vi "George.vi"() -> ()   [LabVIEW 2014]
uses:
  <userlib>/CurtinCode/DataControl.ctl
  <userlib>/CurtinCode/SettingsControl.ctl
  <userlib>/CurtinCode/FilterCtrl.ctl
  <vilib>/sound2/lvsound2.llb/Sound File Info (path).vi
panel:
  out "Average FRF":cluster{dbl, "df":dbl, dbl[]}
  in  "Filter":T1 items=["None", "1 Octave", "1/3 Octave", "1/12 Octave", "Custom"]
  in  "Delete last Run":bool
  out "Average":string
  out "Pts in Ave":u8
  out "selected paths":path[](array[path])
  in  "Open File":bool
  out "Mic Spectrum":cluster{dbl, "df":dbl, dbl[]}(graph)
  out "Alarm":string
  out "Raw Data":T2={"Settings"={"Data Path"=path "", "Time"=timestamp(0 s since 1904-01-01), "Sampling Rate (Hz)"=44800, "Device"=0, "pre-trigger (sec)"=100.0, "length of sample (sec)"=1000.0, "trigger value (V)"=100.0, "Labels"=[], "Cutoffs (sec)"=[], "Freq Bands"=[]}, "Data"=[], "Plot type"=enum."Linear"} {"Settings"."Time" format="%<%H:%M\n%d/%m/%y>T"}
  in  "Tab Control":enum32{"Page 1", "Page 2"}(tab)
  in  "Close Help":bool
  out "Help Text":bool
  in  "Help":bool
  out "version":string="0.1"
  in  "Test":bool
  out "Point":u8(slide) scale=0.0..12.0
  out "Hit":u8(slide) scale=0.0..5.0
  out "current run":string
  in  "Run Conditions":T4={"hits per point"=5, "points per run"=12, "Project Path"=path ""} {"hits per point" items=["1 hit/pt"=1, "5 hits/pt"=5, "10 hits/pt"=10]; "points per run" items=["1 pt/run"=1, "6 pts/run"=6, "12 pts/run"=12]}
  in  "Record":bool
  in  "microphone settings":T5={"resolution"=24, "Sampling rate"=44100, "Sample time"=1.0, "device"=0} {"device" items=["Microphone (High Definition Audio Device)"=0, "DAQmx"=1000]; "resolution" items=["16 bit"=16, "24 bit"=24, "32 bit"=32]; "Sample time" items=["0.5 s"=0.5, "1 s"=1.0]; "Sampling rate" items=["22050 samp/s"=22050, "44100 samp/s"=44100, "48000 samp/s"=48000]}
  out "Filtered FRF":cluster{"Fctr":ext[], "magnitude":dbl[]}[](graph)
  out "Hammer":cluster{i32, dbl, "Data set":dbl[]}(graph)
  out "Microphone":cluster{i32, dbl, "Data set":dbl[]}(graph)
  out "Hammer spectrum":cluster{dbl, "df":dbl, dbl[]}(graph)
  out "Current FRF":cluster{dbl, "df":dbl, dbl[]}(graph)
  out "Live Mic":cluster{i32, dbl, "Data set":dbl[]}(graph)
  # "The Violin Analyzer - version"
  # "Run a test or record an entire run"
  # "See Progess through run"
  # "Set cutoff with green cursors"
  # "Set threshold with purple cursor"
  # "Select Input Device and Settings"
  # "Name Run and Set Run Parameters"
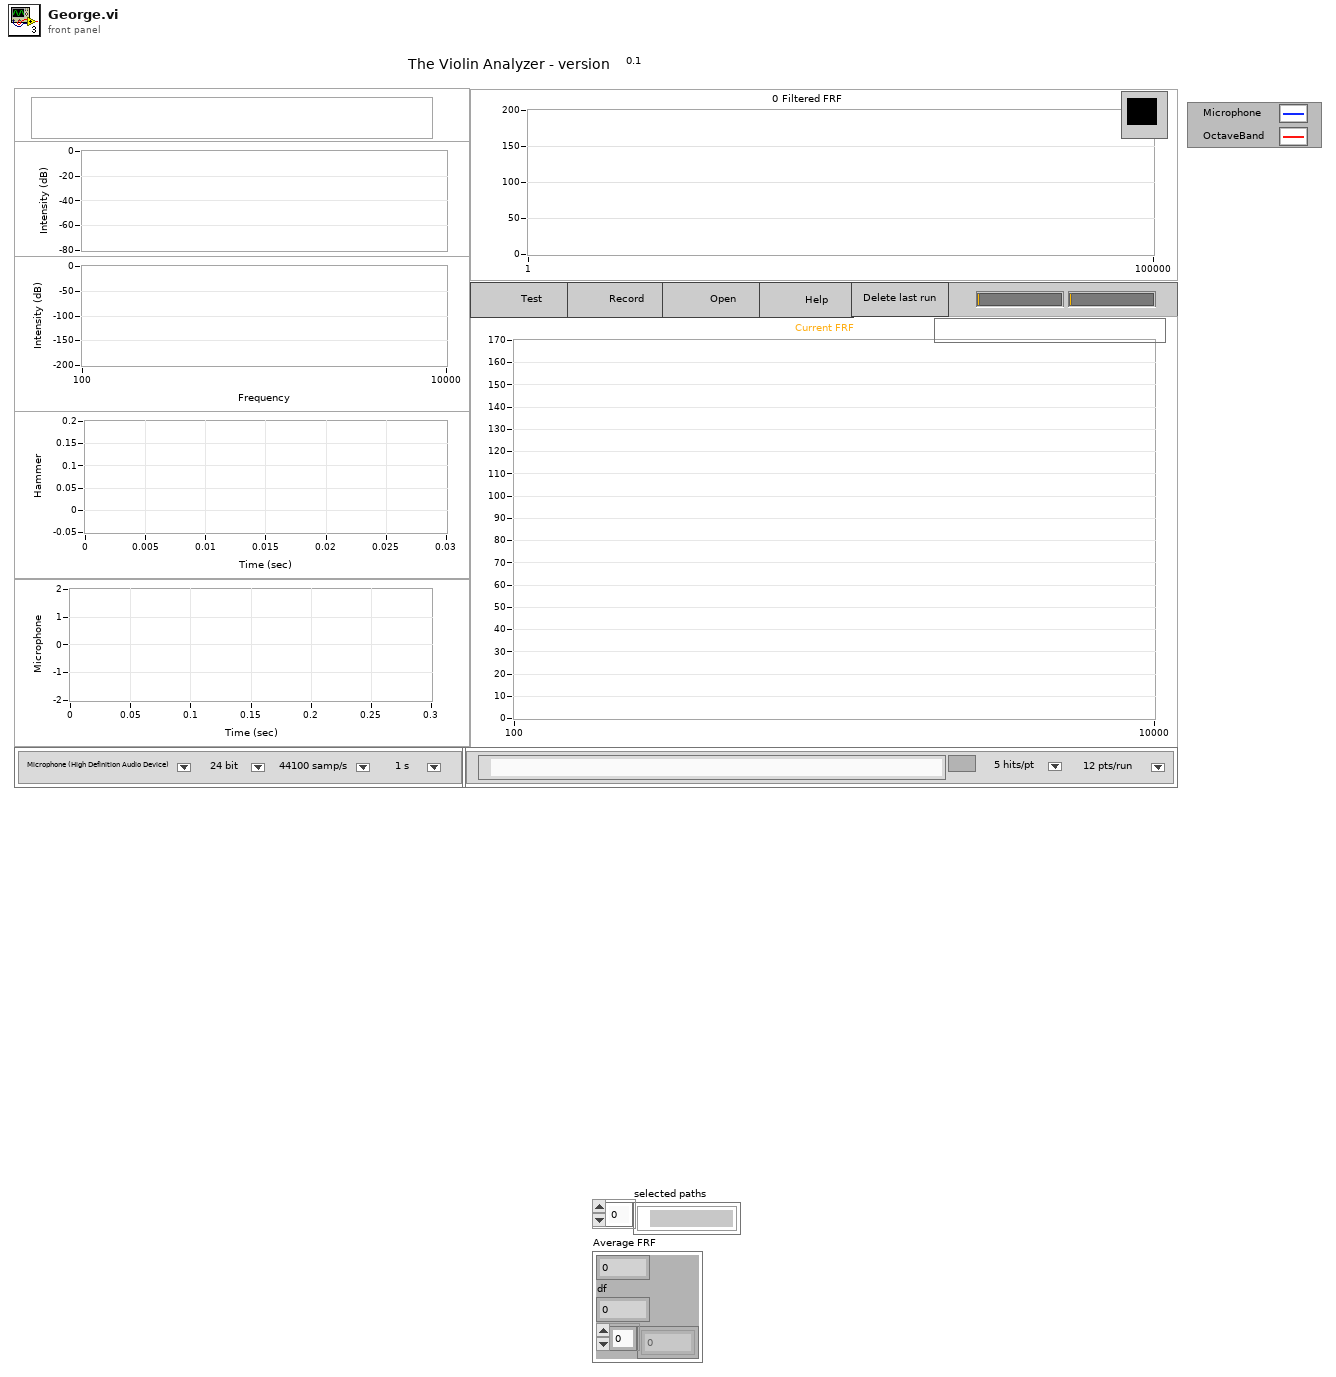
[diagram p1: front panel]
types:
  T1 = typedef "FilterCtrl.ctl" = i8
  T2 = typedef "DataControl.ctl" = cluster{"Settings":T3, "Data":cluster{i32, dbl, "data":dbl[]}[], "Plot type":enum16{"Linear", "log"}}
  T3 = typedef "SettingsControl.ctl" = cluster{"Data Path":path, "Time":timestamp, "Sampling Rate (Hz)":u16, "Device":u16, "pre-trigger (sec)":dbl, "length of sample (sec)":dbl, "trigger value (V)":dbl, "Labels":string[], "Cutoffs (sec)":dbl[], "Freq Bands":dbl[]}
  T4 = cluster{"hits per point":u16, "points per run":u16, "Project Path":path}
  T5 = cluster{"resolution":u16, "Sampling rate":u16, "Sample time":dbl, "device":u16}
  T6 = typedef "AllDataCtrl.ctl" = cluster{"Data Set":T2, "number of samples/ch":i32, "task ID":T7, "error out":errorcluster, "DAQmx task":refnum<k21>}
  T7 = typedef "Sound Input Task ID.ctl" = u32
  T8 = typedef "Sound Data Format.ctl" = cluster{"sample rate (S/s)":dbl, "number of channels":i32, "bits per sample":i32}
  T9 = typedef "LVRangeTypeDef.ctl" = cluster{"Minimum":dbl, "Maximum":dbl, "Increment":dbl, "Minor Increment":dbl, "Start":dbl}
  T10 = typedef "LVStringsAndValuesArrayTypeDef.ctl" = cluster{"String":string, "Value":ext}[]
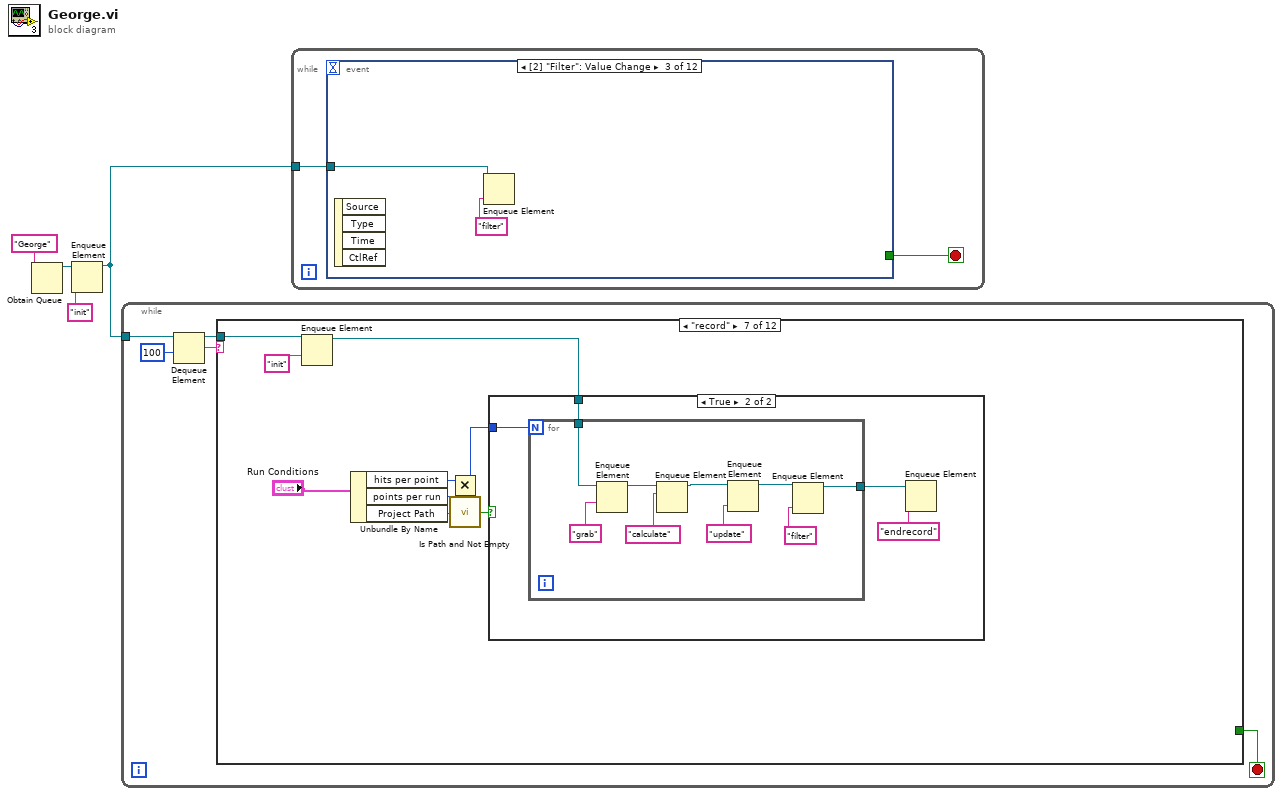
[diagram p0: block diagram]
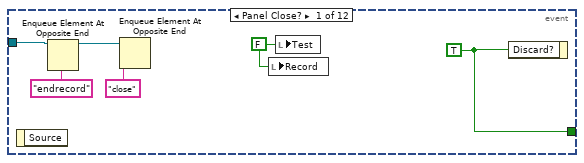
[diagram p2: hidden frame]
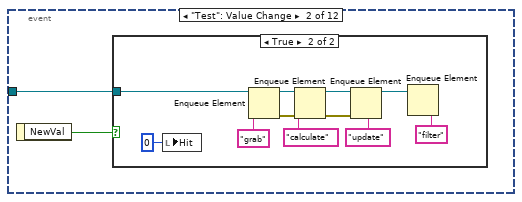
[diagram p3: hidden frame]
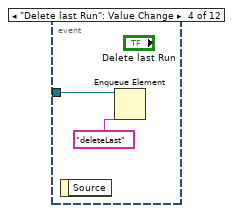
[diagram p5: hidden frame]
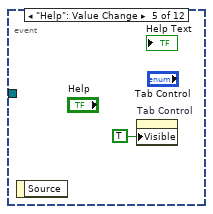
[diagram p6: hidden frame]
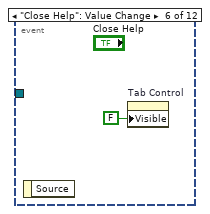
[diagram p7: hidden frame]
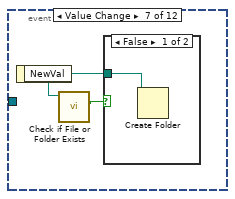
[diagram p8: hidden frame]
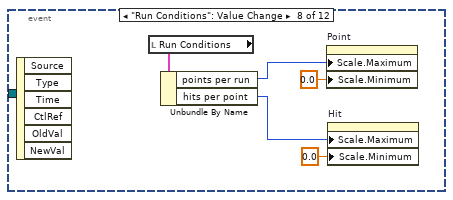
[diagram p10: hidden frame]
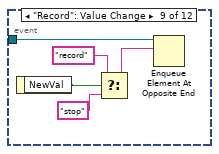
[diagram p11: hidden frame]
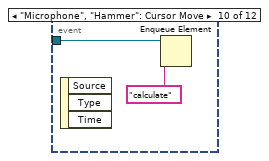
[diagram p12: hidden frame]
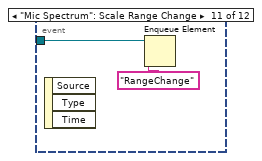
[diagram p13: hidden frame]
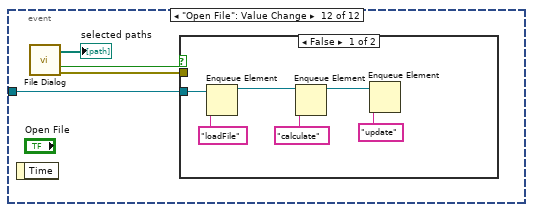
[diagram p14: hidden frame]
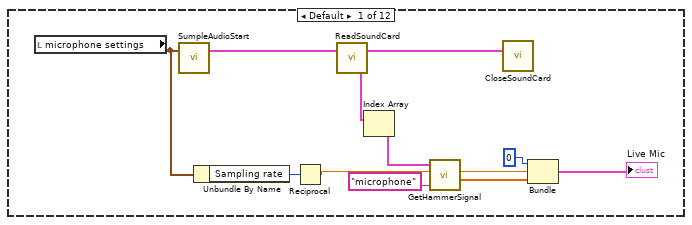
[diagram p16: hidden frame]
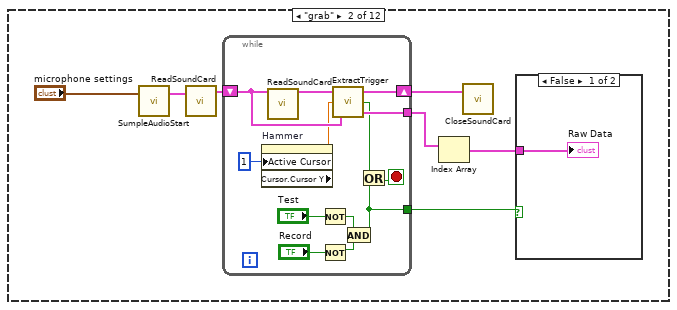
[diagram p17: hidden frame]
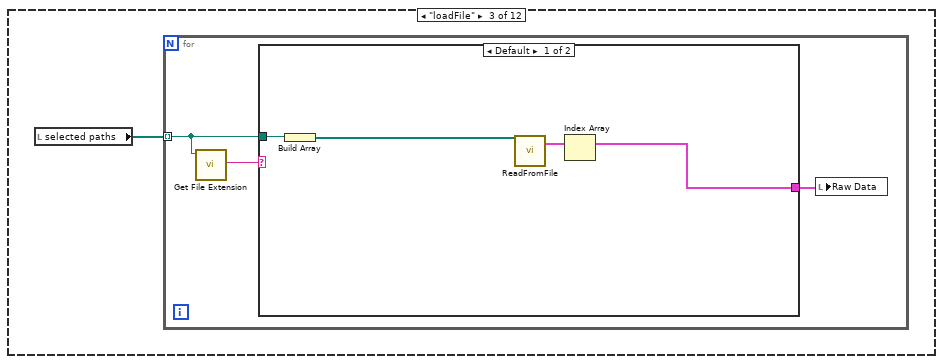
[diagram p19: hidden frame]
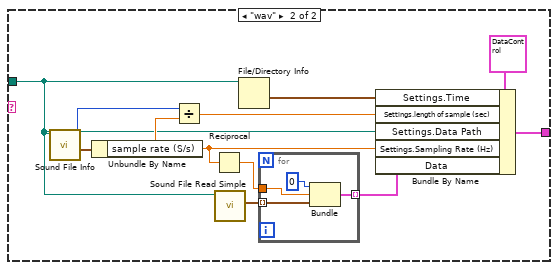
[diagram p20: hidden frame]
diagram:
  w4 = "George" ("name (unnamed)")
  n1 = Obtain Queue(name (unnamed)=w4, element data type=w4) -> (queue out=w3:refnum<queue>)  [unwired: 3 in, 2 out]
  n2 = Enqueue Element(queue=w3, element="init") -> (queue out=w1:refnum<queue>)  [unwired: 2 in, 2 out]
  n3 = while {
    tunnel: w1 -> [w9]
    stop <- w7 stop-if-true
    n4 = Dequeue Element(queue=w9, timeout in ms (-1)=100) -> (queue out=w6:refnum<queue>, element=w8:string)  [unwired: 1 in, 2 out]
    n5 = case shown="\"record\"" w8 {
      tunnel: [_ _ _ _ _ _ _ _ _ _ _ TRUE ("Discard?")] -> w7
      tunnel: w6 -> [_ _ _ _ _ _ w156 _ w178 _ w225 _]
      frame Default {
        n6 = local read "microphone settings"() -> (w12:T5)
        n7 = call <userlib>:"SumpleAudioStart.vi"("microphone settings"=w12) -> ("All Info"=w20:T6)  [unwired: 2 in]
        n8 = Unbundle By Name(w12) -> ("Sampling rate"=w13:u16)
        n9 = Reciprocal(x=w13) -> (1/x=w11:dbl)
        n10 = call <userlib>:"ReadSoundCard.vi"("All Info"=w20) -> ("Data Set"=w18:T2[], "All Info"=w19:T6)  [unwired: 1 in]
        n11 = Index Array(array=w18) -> (element=w17:T2)  [unwired: 1 in]
        n12 = call <userlib>:"GetHammerSignal.vi"("column"="microphone", "Data Set"=w17) -> ("Data set"=w14:dbl[])  [unwired: 1 in, 2 out]
        n13 = call <userlib>:"CloseSoundCard.vi"("All Info"=w19) -> ()  [unwired: 3 in]
        n14 = Bundle(0, w11, "Data set"=w14) -> (→"Live Mic":cluster{i32, dbl, "Data set":dbl[]})  [unwired: 1 in]
      }
      frame "grab" {
        n15 = call <userlib>:"SumpleAudioStart.vi"("microphone settings"="microphone settings") -> ("All Info"=w26:T6)  [unwired: 2 in]
        n16 = call <userlib>:"ReadSoundCard.vi"("All Info"=w26) -> ("All Info"=w25:T6)  [unwired: 1 in, 1 out]
        n17 = while {
          shift-right: [w41] -> w27
          shift-left: w25 -> [w39]
          tunnel: [w38] -> w23
          tunnel: [w29] -> w21
          stop <- w33 stop-if-true
          n18 = property on="Hammer" class="WFGraph (strict)"("Active Cursor"=u32 1) -> ("Cursor.Cursor Y"=w36:dbl)  [unwired: 2 in, 2 out]
          n19 = call <userlib>:"ReadSoundCard.vi"("All Info"=w39) -> ("All Info"=w40:T6)  [unwired: 1 in, 1 out]
          n20 = Not(x="Test") -> (.not. x?=w30:bool)
          n21 = Not(x="Record") -> (.not. x?=w31:bool)
          n22 = call <userlib>:"ExtractTrigger.vi"(3:"All Info"=w39, "Trigger"=w36, 5:"All Info"=w40) -> ("Data Set"=w38:T2[], "Trigger?"=w35:bool, "All Info"=w41:T6)
          n23 = And(x=w30, y=w31) -> (x .and. y?=w29:bool)
          n24 = Or(x=w35, y=w29) -> (x .or. y?=w33:bool)
        }
        n25 = Index Array(array=w23) -> (element=w22:T2)  [unwired: 1 in]
        n26 = call <userlib>:"CloseSoundCard.vi"("All Info"=w27) -> ()  [unwired: 3 in]
        n27 = case shown="False" w21 {
          tunnel: w22 -> [w28 _]
          frame False {
            "Raw Data" <- w28
          }
          frame True {
          }
        }
      }
      frame "loadFile" {
        n28 = local read "selected paths"() -> (w42:path[])
        n29 = for {
          tunnel: w42 -> [w44] mode=indexing
          n30 = call <vilib>:"Get File Extension.vi"("file"=w44) -> ("lowercase file extension"=w43:string)  [unwired: 7 in, 3 out]
          n31 = case shown="Default" w43 {
            tunnel: [w46 w52] -> w45
            tunnel: w44 -> [w49 w50]
            frame Default {
              n32 = Build Array(w49) -> (w48:path[])
              n33 = call <userlib>:"ReadFromFile.vi"("File paths"=w48) -> ("Data Sets"=w47:T2[])  [unwired: 1 in, 1 out]
              n34 = Index Array(array=w47) -> (element=w46:T2)  [unwired: 1 in]
            }
            frame "wav" {
              n35 = call-poly <vilib>:"Sound File Info.vi"("path"=w50) -> ("sound format"=w59:T8, "total number of samples/ch"=w55:u32)  [unwired: 7 in, 2 out]
              n36 = Unbundle By Name(w59) -> ("sample rate (S/s)"=w56:dbl)
              n37 = Divide(x=w55, y=w56) -> (x/y=w54:dbl)
              n38 = Reciprocal(x=w56) -> (1/x=w60:dbl)
              n39 = call <vilib>:"Sound File Read Simple.vi"("path"=w50) -> ("data"=w57:waveform(dbl)[])  [unwired: 7 in, 3 out]
              n40 = File/Directory Info(path=w50) -> (last mod=w53:timestamp)  [unwired: 1 in, 6 out]
              n41 = for {
                tunnel: w60 -> [w63]
                tunnel: [w62] -> w58 mode=indexing
                tunnel: w57 -> [w61] mode=indexing
                n42 = Bundle(0, w63, "data"=w61) -> (w62:cluster{i32, dbl, "data":waveform(dbl)})  [unwired: 1 in]
              }
              n43 = Bundle By Name(cluster=T2 {"Settings"={"Data Path"=path "", "Time"=timestamp(0 s since 1904-01-01), "Sampling Rate (Hz)"=44800, "Device"=0, "pre-trigger (sec)"=100.0, "length of sample (sec)"=1000.0, "trigger value (V)"=100.0, "Labels"=[], "Cutoffs (sec)"=[], "Freq Bands"=[]}, "Data"=[], "Plot type"=enum."Linear"} ("Data Set"), "Settings.Time"=w53, "Settings.length of sample (sec)"=w54, "Settings.Data Path"=w50, "Settings.Sampling Rate (Hz)"=w56, "Data"=w58) -> (w52:T2)
            }
          }
          n44 = local write "Raw Data"(w45) -> ()
        }
      }
      frame "calculate" {
        n45 = property on="Hammer" class="WFGraph (strict)"("Active Cursor"=u32 0) -> ("Cursor.Cursor X"=w69:dbl)  [unwired: 2 in, 2 out]
        n46 = property on="Microphone" class="WFGraph (strict)"("Active Cursor"=u32 0) -> ("Cursor.Cursor X"=w70:dbl)  [unwired: 2 in, 2 out]
        n47 = Build Array(w70, w69) -> (w71:dbl[])
        n48 = local read "Raw Data"() -> (w92:T2)
        n49 = Bundle By Name(cluster=w92, "Settings.Cutoffs (sec)"=w71) -> (w68:T2)
        n50 = local read "microphone settings"() -> (w91:T5)
        n51 = Unbundle By Name(w91) -> ("Sampling rate"=w90:u16)
        n52 = local write "Raw Data"(w68) -> ()
        n53 = Reciprocal(x=w90) -> (1/x=w88:dbl)
        n54 = call <userlib>:"GetHammerSignal.vi"("column"="hammer", "Data Set"=w68) -> ("Cutoff"=w94:dbl, "Data set"=w86:dbl[], "time between samples"=w93:dbl)  [unwired: 1 in]
        n55 = call <userlib>:"GetHammerSignal.vi"("column"="microphone", "Data Set"=w68) -> ("Cutoff"=w96:dbl, "Data set"=w81:dbl[], "time between samples"=w97:dbl)  [unwired: 1 in]
        n56 = Bundle(0, w88, "Data set"=w86) -> (→"Hammer":cluster{i32, dbl, "Data set":dbl[]})  [unwired: 1 in]
        n57 = call <userlib>:"FourierTransform.vi"("Cutoff (s)"=w94, "Time Data"=w86, "time per sample"=w93) -> ("Spectrum"=→"Hammer spectrum":cluster{dbl, "df":dbl, dbl[]}, "FFT"=w67:cluster{dbl, "df":dbl, "FFT {X}":cdb[]})
        n58 = Bundle(0, w88, "Data set"=w81) -> (→"Microphone":cluster{i32, dbl, "Data set":dbl[]})  [unwired: 1 in]
        n59 = call <userlib>:"FourierTransform.vi"("Cutoff (s)"=w96, "Time Data"=w81, "time per sample"=w97) -> ("Spectrum"=→"Mic Spectrum":cluster{dbl, "df":dbl, dbl[]}, "FFT"=w66:cluster{dbl, "df":dbl, "FFT {X}":cdb[]})
        n60 = Greater?(x=w81, y=0.99) -> (0:w83:bool[])
        n61 = Greater?(x=w86, y=0.99) -> (0:w84:bool[])
        n62 = call <userlib>:"FindFRF.vi"("Microphone FFT"=w66, "Hammer FFT"=w67) -> ("Current FRF"=→"Current FRF":cluster{dbl, "df":dbl, dbl[]})  [unwired: 1 out]
        n63 = Or Array Elements(Boolean array=w83) -> (logical OR=w80:bool)
        n64 = Or Array Elements(Boolean array=w84) -> (logical OR=w77:bool)
        n65 = Select(t="Microphone Signal Clipped", s=w80, f="") -> (s? t:f=w76:string)
        n66 = Select(t="Hammer Signal Clipped", s=w77, f=w76) -> (s? t:f=w74:string)
        n67 = local write "Alarm"(w74) -> ()
      }
      frame "RangeChange" {
        n68 = property on="Mic Spectrum" class="WFGraph (strict)"() -> (error out=w104:errorcluster, "XScale.Range"=w103:T9)  [unwired: 2 in, 1 out]
        n69 = property on="Hammer spectrum" class="WFGraph (strict)"(error in=w104, "XScale.Range"=w103) -> ()  [unwired: 1 in, 2 out]
      }
      frame "init" {
        w105 = FALSE ("Test")
        w130 = u8 0 ("% done for run")
        w111 = "" ("current run")
        n70 = local read "Run Conditions"() -> (w107:T4)
        n71 = Unbundle By Name(w107) -> ("points per run"=w109:u16, "hits per point"=w106:u16)
        n72 = flat-sequence {
          tunnel: [w131] -> _
          frame #0 {
            n73 = control-ref of="device"() -> (w138:refnum<vi>)
            n74 = call <vilib>:"InitializeInputDeviceRing.vi"("Device Refnum"=w138) -> ("error out"=w137:errorcluster)  [unwired: 1 in, 13 out]
            n75 = property class="Ring (strict)"(reference=w138, error in=w137) -> (reference out=w133:refnum<vi>, error out=w132:errorcluster, "Strings And Values []"=w136:T10)
            n76 = Build Array (concatenate)(w136, cluster{"String":string, "Value":i32} {"String"="DAQmx", "Value"=1000}) -> (w134:T10)
            n77 = property class="Ring (strict)"(reference=w133, error in=w132, "Strings And Values []"=w134) -> (error out=w131:errorcluster)  [unwired: 1 out]
          }
        }
        n78 = property on="Point" class="Slide (strict)"("Scale.Maximum"=w109, "Scale.Minimum"=0.0 ("Scale.Range:Minimum")) -> ()  [unwired: 2 in, 2 out]
        n79 = property on="Hit" class="Slide (strict)"("Scale.Maximum"=w106, "Scale.Minimum"=0.0 ("Scale.Range:Minimum")) -> ()  [unwired: 2 in, 2 out]
        n80 = property on="Tab Control" class="TabCtl (strict)"("Visible"=FALSE) -> ()  [unwired: 2 in, 2 out]
        n81 = local write "Record"(w105) -> ()
        n82 = local write "current run"(w111) -> ()
        n83 = local write "Test"(w105) -> ()
        n84 = local write "Average"(w111) -> ()
        n85 = property on="Hammer" class="WFGraph (strict)"("Active Cursor"=u32 1) -> ("Cursor.Cursor Y"=w114:dbl, "YScale.Maximum"=w112:dbl)  [unwired: 2 in, 2 out]
        n86 = property on="Hammer" class="WFGraph (strict)"("Active Cursor"=u32 0) -> ("Cursor.Cursor X"=w115:dbl, "XScale.Maximum"=w113:dbl)  [unwired: 2 in, 2 out]
        n87 = property on="Microphone" class="WFGraph (strict)"("Active Cursor"=u32 0) -> ("Cursor.Cursor X"=w127:dbl, "XScale.Maximum"=w126:dbl)  [unwired: 2 in, 2 out]
        n88 = In Range and Coerce(upper limit=0.0, x=w114, lower limit=w112) -> (In Range?=w117:bool)  [unwired: 1 out]
        n89 = In Range and Coerce(upper limit=0.0, x=w115, lower limit=w113) -> (In Range?=w118:bool)  [unwired: 1 out]
        n90 = In Range and Coerce(upper limit=0.0, x=w127, lower limit=w126) -> (In Range?=w124:bool)  [unwired: 1 out]
        n91 = And(x=w118, y=w117) -> (x .and. y?=w116:bool)
        n92 = case shown="False" w124 {
          frame False {
            n93 = property on="Microphone" class="WFGraph (strict)"("Active Cursor"=u32 0, "Cursor.Cursor X"=0.2 ("Cursor.Cursor Position:Cursor X")) -> ()  [unwired: 2 in, 2 out]
          }
          frame True {
          }
        }
        n94 = case shown="False" w116 {
          tunnel: w113 -> [w144 _]
          tunnel: w112 -> [w140 _]
          frame False {
            n95 = Divide(x=w144, y=2.0 ("upper limit")) -> (x/y=w142:dbl)
            n96 = Divide(x=w140, y=2.0 ("upper limit")) -> (x/y=w139:dbl)
            n97 = property on="Hammer" class="WFGraph (strict)"("Active Cursor"=u32 0, "Cursor.Cursor X"=w142, "Active Cursor"=u32 1, "Cursor.Cursor Y"=w139) -> ()  [unwired: 2 in, 2 out]
          }
          frame True {
          }
        }
        "Point" <- w130
        "Hit" <- w130
        "version" <- "0.1" ("version")
        "Alarm" <- w111
      }
      frame "record" {
        n98 = Enqueue Element(queue=w156, element="init") -> (queue out=w150:refnum<queue>)  [unwired: 2 in, 2 out]
        n99 = Unbundle By Name("Run Conditions") -> ("hits per point"=w153:u16, "points per run"=w152:u16, "Project Path"=w155:path)
        n100 = Multiply(x=w153, y=w152) -> (x*y=w151:u16)
        n101 = call <vilib>:"Is Path and Not Empty.vi"("path"=w155) -> ("Is Path and Not Empty?"=w154:bool)  [unwired: 4 in]
        n102 = case shown="True" w154 {
          tunnel: w151 -> [_ w163]
          tunnel: w150 -> [_ w162]
          frame False {
            n103 = One Button Dialog(message="Please choose a folder for data") -> ()  [unwired: 1 in, 1 out]
            n104 = local write "Record"(FALSE ("Record")) -> ()
          }
          frame True {
            n105 = for {
              N: w163 -> [_]
              tunnel: w162 -> [w171]
              tunnel: [w164] -> w161
              n106 = Enqueue Element(queue=w171, element="grab") -> (queue out=w169:refnum<queue>)  [unwired: 2 in, 2 out]
              n107 = Enqueue Element(queue=w169, element="calculate") -> (queue out=w168:refnum<queue>)  [unwired: 2 in, 2 out]
              n108 = Enqueue Element(queue=w168, element="update") -> (queue out=w165:refnum<queue>)  [unwired: 2 in, 2 out]
              n109 = Enqueue Element(queue=w165, element="filter") -> (queue out=w164:refnum<queue>)  [unwired: 2 in, 2 out]
            }
            n110 = Enqueue Element(queue=w161, element="endrecord") -> ()  [unwired: 2 in, 3 out]
          }
        }
      }
      frame "endrecord" {
        w173 = "" ("Alarm")
        n111 = local write "Test"(FALSE ("Test")) -> ()
        n112 = local write "Record"(FALSE ("Test")) -> ()
        n113 = local write "Average"(w173) -> ()
        n114 = local write "Alarm"(w173) -> ()
      }
      frame "update" {
        n115 = local read "Test"() -> (w179:bool)
        n116 = local read "Run Conditions"() -> (w193:T4)
        n117 = Unbundle By Name(w193) -> ("hits per point"=w181:u16, "Project Path"=w191:path)
        n118 = local read "Hit"() -> (w184:u8)
        n119 = local read "Point"() -> (w182:u8)
        n120 = case shown="True" w179 {
          tunnel: w178 -> [_ w205]
          frame False {
          }
          frame True {
            n121 = Enqueue Element(queue=w205, element="grab") -> (queue out=w204:refnum<queue>, error out=w203:errorcluster)  [unwired: 2 in, 1 out]
            n122 = Enqueue Element(queue=w204, element="calculate", error in (no error)=w203) -> (queue out=w202:refnum<queue>, error out=w201:errorcluster)  [unwired: 1 in, 1 out]
            n123 = Enqueue Element(queue=w202, element="update", error in (no error)=w201) -> (queue out=w197:refnum<queue>, error out=w196:errorcluster)  [unwired: 1 in, 1 out]
            n124 = Enqueue Element(queue=w197, element="filter", error in (no error)=w196) -> ()  [unwired: 1 in, 3 out]
          }
        }
        n125 = Increment(x=w184) -> (x+1=w177:u8)
        "Pts in Ave" <- w177
        n126 = Quotient & Remainder(x=w177, y=w181) -> (x-y*floor(x/y)=w187:u16, floor(x/y)=w195:u16)
        n127 = Format Into String(format string="SoundFile_%02d_%02d.dat", w182, w184) -> (resulting string=w189:string)  [unwired: 2 in, 1 out]
        "current run" <- w189
        n128 = Format Into String(format string="%d/%d hit (point %d)", w177, w181, w182) -> (resulting string=→"Average":string)  [unwired: 2 in, 1 out]
        n129 = Add(x=w195, y=w182) -> (x+y=w194:u16)
        n130 = local write "Point"(w194) -> ()
        n131 = local write "Hit"(w187) -> ()
        n132 = Build Path(base path=w191, name or relative path=w189) -> (appended path=w190:path)
        n133 = local read "Current FRF"() -> (w186:cluster{dbl, "df":dbl, dbl[]})
        n134 = local read "Average FRF"() -> (w188:cluster{dbl, "df":dbl, dbl[]})
        n135 = local read "Record"() -> (w180:bool)
        n136 = case shown="True" w180 {
          tunnel: w190 -> [_ w207]
          frame False {
          }
          frame True {
            n137 = local read "Raw Data"() -> (w211:T2)
            n138 = Unbundle By Name(w211) -> ("Settings"=w210:T3, "Data"=w209:cluster{i32, dbl, "data":dbl[]}[])
            n139 = for {
              tunnel: w209 -> [w213] mode=indexing
              tunnel: [w212] -> w208 mode=indexing
              n140 = Unbundle(w213) -> ("data"=w212:dbl[])  [unwired: 2 out]
            }
            n141 = call <userlib>:"SaveToFile.vi"("Data"=w208, "Settings"=w210, "Path In"=w207) -> ()  [unwired: 2 in, 1 out]
          }
        }
        n142 = case shown="Default" w184 {
          selector: w184 -> [w216 _]
          tunnel: w188 -> [w220 _]
          tunnel: [w214 w221] -> w176
          tunnel: w186 -> [w218 w221]
          frame Default {
            n143 = Multiply(x=w220, y=w216) -> (x*y=w219:cluster{dbl, "df":dbl, dbl[]})
            n144 = Add(x=w218, y=w219) -> (x+y=w217:cluster{dbl, "df":dbl, dbl[]})
            n145 = Increment(x=w216) -> (x+1=w215:u8)
            n146 = Divide(x=w217, y=w215) -> (x/y=w214:cluster{dbl, "df":dbl, dbl[]})
          }
          frame 0 {
          }
        }
        "Average FRF" <- w176
      }
      frame "filter" {
        n147 = local read "Average FRF"() -> (w222:cluster{dbl, "df":dbl, dbl[]})
        n148 = call <userlib>:"OctaveBandAnalysis.vi"("Filter"="Filter", "Current FRF"=w222) -> ("FRF Bands 2"=→"Filtered FRF":cluster{"Fctr":ext[], "magnitude":dbl[]}[])  [unwired: 1 in]
      }
      frame "stop" {
        n149 = Flush Queue(queue=w225) -> ()  [unwired: 1 in, 3 out]
      }
      frame "close" {
        n150 = local write "Alarm"("" ("Alarm")) -> ()
      }
    }
  }
  n151 = while {
    tunnel: w1 -> [w228]
    stop <- w229 stop-if-true
    n152 = event shown="[2] \"Filter\": Value Change" {
      selector: _ -> [_ _ _ _ _ _ _ _ _ _ _ _]
      dyn-events: _ -> [_ _ _ _ _ _ _ _ _ _ _ _]
      timeout: _ -> [_ _ _ _ _ _ _ _ _ _ _ _]
      tunnel: [w235 _ _ _ _ _ _ _ _ _ _ _] -> w229
      tunnel: w228 -> [w232 w237 w249 w251 _ _ _ _ w267 w268 w270 w274]
      event Panel Close? {
        w230 = FALSE ("Test")
        w235 = TRUE ("Discard?")
        n153 = event-data() -> ()  [unwired: 1 in, 1 out]
        n154 = Enqueue Element At Opposite End(queue=w232, element="endrecord") -> (queue out=w231:refnum<queue>)  [unwired: 2 in, 2 out]
        n155 = Enqueue Element At Opposite End(queue=w231, element="close") -> ()  [unwired: 2 in, 3 out]
        n156 = local write "Record"(w230) -> ()
        n157 = local write "Test"(w230) -> ()
        n158 = event-data("Discard?"=w235) -> ()  [unwired: 1 in, 1 out]
      }
      event "Test": Value Change {
        n159 = event-data() -> ("NewVal"=w236:bool)  [unwired: 1 in]
        n160 = case shown="True" w236 {
          tunnel: w237 -> [_ w247]
          frame False {
          }
          frame True {
            n161 = local write "Hit"(u8 0 ("Hit")) -> ()
            n162 = Enqueue Element(queue=w247, element="grab") -> (queue out=w245:refnum<queue>, error out=w244:errorcluster)  [unwired: 2 in, 1 out]
            n163 = Enqueue Element(queue=w245, element="calculate", error in (no error)=w244) -> (queue out=w241:refnum<queue>, error out=w242:errorcluster)  [unwired: 1 in, 1 out]
            n164 = Enqueue Element(queue=w241, element="update", error in (no error)=w242) -> (queue out=w239:refnum<queue>)  [unwired: 1 in, 2 out]
            n165 = Enqueue Element(queue=w239, element="filter") -> ()  [unwired: 2 in, 3 out]
          }
        }
      }
      event Value Change {
        n166 = event-data() -> ()  [unwired: 1 in, 4 out]
        n167 = Enqueue Element(queue=w249, element="filter") -> ()  [unwired: 2 in, 3 out]
      }
      event "Delete last Run": Value Change {
        n168 = event-data() -> ()  [unwired: 1 in, 1 out]
        n169 = Enqueue Element(queue=w251, element="deleteLast") -> ()  [unwired: 2 in, 3 out]
      }
      event "Help": Value Change {
        n170 = event-data() -> ()  [unwired: 1 in, 1 out]
        n171 = property on="Tab Control" class="TabCtl (strict)"("Visible"=TRUE) -> ()  [unwired: 2 in, 2 out]
      }
      event "Close Help": Value Change {
        n172 = event-data() -> ()  [unwired: 1 in, 1 out]
        n173 = property on="Tab Control" class="TabCtl (strict)"("Visible"=FALSE) -> ()  [unwired: 2 in, 2 out]
      }
      event "Run Conditions.Project Path": Value Change {
        n174 = event-data() -> ("NewVal"=w255:path)  [unwired: 1 in]
        n175 = call <vilib>:"Check if File or Folder Exists.vi"("path"=w255) -> ("file or folder exists?"=w256:bool)  [unwired: 8 in, 2 out]
        n176 = case shown="False" w256 {
          tunnel: w255 -> [w257 _]
          frame False {
            n177 = Create Folder(path (use dialog)=w257) -> ()  [unwired: 2 in, 3 out]
          }
          frame True {
          }
        }
      }
      event "Run Conditions": Value Change {
        n178 = event-data() -> ()  [unwired: 1 in, 6 out]
        n179 = local read "Run Conditions"() -> (w261:T4)
        n180 = Unbundle By Name(w261) -> ("points per run"=w259:u16, "hits per point"=w262:u16)
        n181 = property on="Point" class="Slide (strict)"("Scale.Maximum"=w259, "Scale.Minimum"=0.0 ("Scale.Range:Minimum")) -> ()  [unwired: 2 in, 2 out]
        n182 = property on="Hit" class="Slide (strict)"("Scale.Maximum"=w262, "Scale.Minimum"=0.0 ("Scale.Range:Minimum")) -> ()  [unwired: 2 in, 2 out]
      }
      event "Record": Value Change {
        n183 = event-data() -> ("NewVal"=w263:bool)  [unwired: 1 in]
        n184 = Select(t="record" ("element"), s=w263, f="stop" ("element")) -> (s? t:f=w265:string)
        n185 = Enqueue Element At Opposite End(queue=w267, element=w265) -> ()  [unwired: 2 in, 3 out]
      }
      event "Microphone", "Hammer": Cursor Move {
        n186 = event-data() -> ()  [unwired: 1 in, 3 out]
        n187 = Enqueue Element(queue=w268, element="calculate") -> ()  [unwired: 2 in, 3 out]
      }
      event "Mic Spectrum": Scale Range Change {
        n188 = event-data() -> ()  [unwired: 1 in, 3 out]
        n189 = Enqueue Element(queue=w270, element="RangeChange") -> ()  [unwired: 2 in, 3 out]
      }
      event "Open File": Value Change {
        n190 = event-data() -> ()  [unwired: 1 in, 1 out]
        n191 = call "File Dialog"() -> ("selected paths"=→"selected paths":path[], "cancelled"=w275:bool, "error out"=w273:errorcluster)  [unwired: 12 in, 1 out]
        n192 = case shown="False" w275 {
          tunnel: w274 -> [w279 _]
          tunnel: w273 -> [_ _]
          frame False {
            n193 = Enqueue Element(queue=w279, element="loadFile") -> (queue out=w278:refnum<queue>)  [unwired: 2 in, 2 out]
            n194 = Enqueue Element(queue=w278, element="calculate") -> (queue out=w276:refnum<queue>)  [unwired: 2 in, 2 out]
            n195 = Enqueue Element(queue=w276, element="update") -> ()  [unwired: 2 in, 3 out]
          }
          frame True {
          }
        }
      }
    }
  }
